vi "select elements to create channels for.vi"(8 "error in":errorcluster, 10 "allowable channels":i32[](array[numeric]), 11 "assembly definition":T1) -> (0 "error out":errorcluster, 1 "cancelled?":bool, 2 "channels to create":i32[](array[numeric]), 3 "base channame":string, 5 "create tags":bool)   [LabVIEW 2013, in "EthernetIP editor node.lvclass"]
uses:
  EthernetIP editor node.lvclass
  configuration/assembly definition.ctl
  configuration/assembly type.ctl
  <vilib>/NI/Tag Bus/tag/Data Type.ctl
  configuration/EthernetIP configuration.lvclass
  <vilib>/NI/Tag Bus/tag/tag descriptor.lvclass
panel:
  in  "Also Create Tags?":bool
  in  "cancel":bool
  in  "Base Name":string
  in  "OK":bool
  in  "Remove":bool
  in  "Add":bool
  in  "Channels to Configure":i32[](listbox)
  in  "Allowable Channels":i32[](listbox)
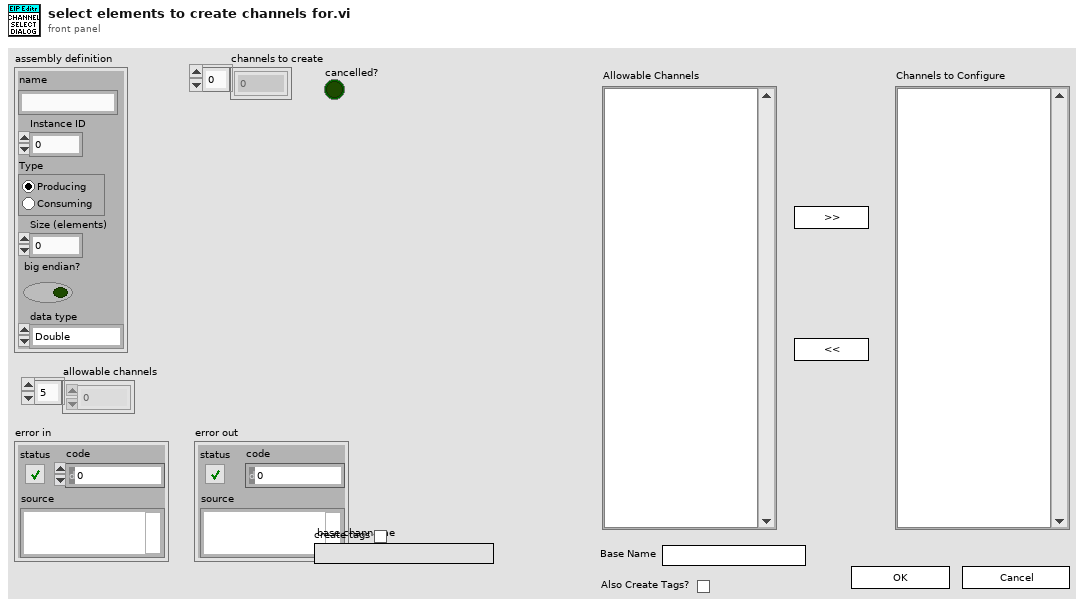
[diagram p1: front panel]
types:
  T1 = typedef "EthernetIP configuration.lvclass/assembly definition.ctl" = cluster{"name":string, "Instance ID":u32, "Type":T2, "Size (elements)":u32, "big endian?":bool, "data type":T3}
  T2 = typedef "EthernetIP configuration.lvclass/assembly type.ctl" = enum32{"Producing", "Consuming"}
  T3 = typedef "tag bus.lvlib/tag descriptor.lvclass/Data Type.ctl" = enum16{"Double", "Single", "I64", "I32", "I16", "I8", "U64", "U32", "U16", "U8", "Boolean", "String", "Array of Double", "Array of Single", "Array of I64", "Array of I32", "Array of I16", "Array of I8", "Array of U64", "Array of U32", "Array of U16", "Array of U8", "Array of Boolean", "Array of String"}
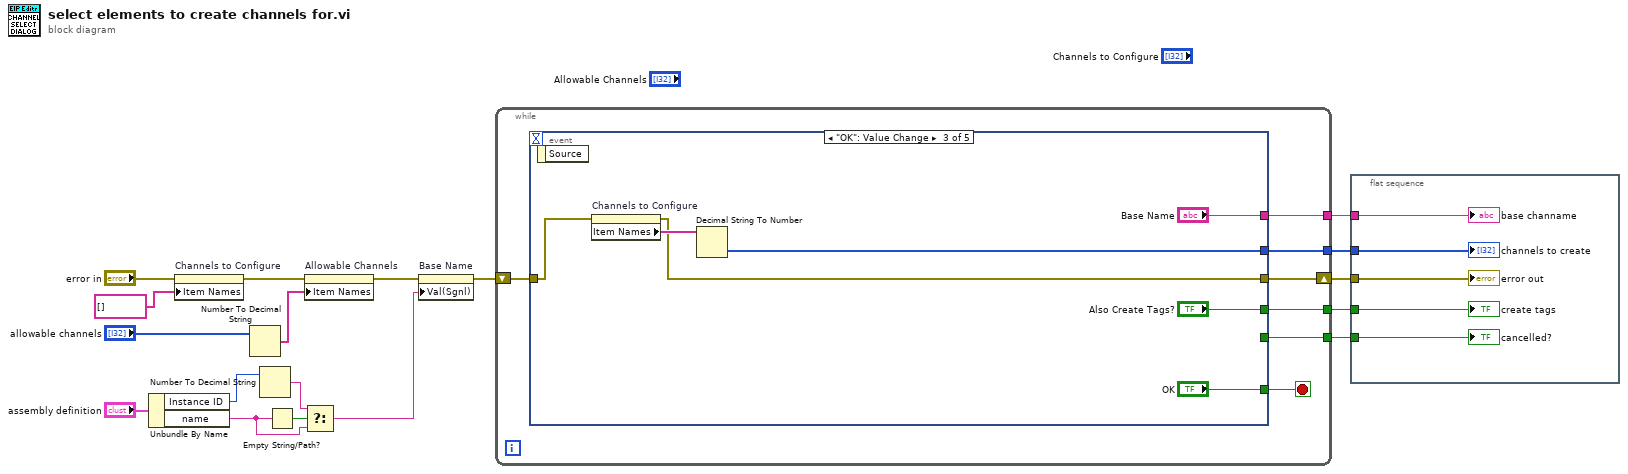
[diagram p0: block diagram]
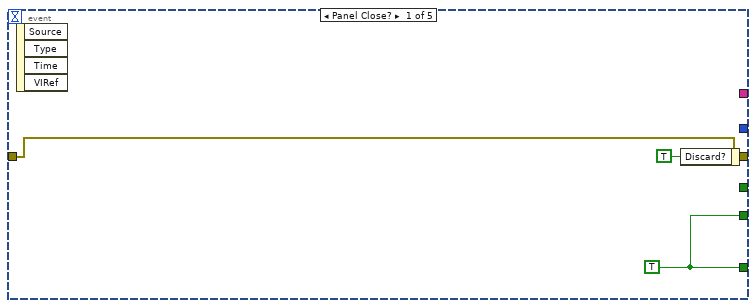
[diagram p2: hidden frame]
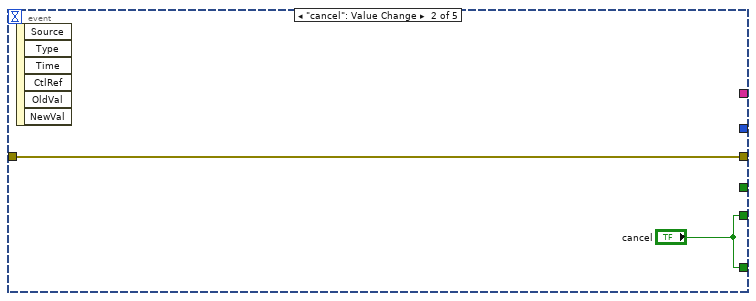
[diagram p3: hidden frame]
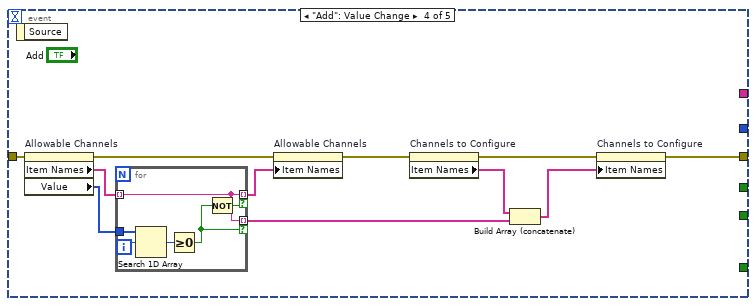
[diagram p4: hidden frame]
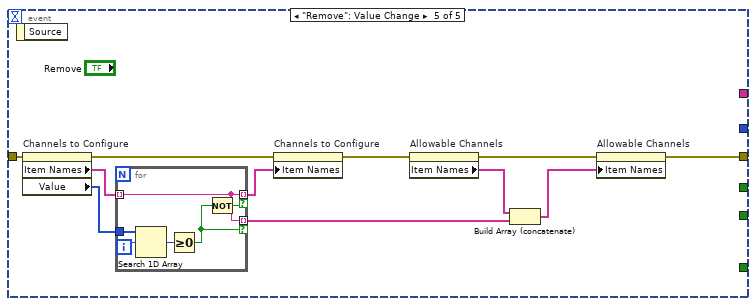
[diagram p5: hidden frame]
diagram:
  n1 = Unbundle By Name("assembly definition") -> ("Instance ID"=w8:u32, "name"=w9:string)
  n2 = property on="Channels to Configure" class="LstBox (strict)"(error in="error in", "Item Names"=string[] []) -> (error out=w4:errorcluster)  [unwired: 1 in, 1 out]
  n3 = Number To Decimal String(number="allowable channels") -> (decimal integer string=w15:string[])  [unwired: 1 in]
  n4 = Number To Decimal String(number=w8) -> (decimal integer string=w7:string)  [unwired: 1 in]
  n5 = Empty String/Path?(string/path=w9) -> (empty?=w10:bool)
  n6 = property on="Allowable Channels" class="LstBox (strict)"(error in=w4, "Item Names"=w15) -> (error out=w12:errorcluster)  [unwired: 1 in, 1 out]
  n7 = Select(t=w7, s=w10, f=w9) -> (s? t:f=w6:string)
  n8 = property on="Base Name" class="Str"(error in=w12, "Val(Sgnl)"=w6) -> (error out=w11:errorcluster)  [unwired: 1 in, 1 out]
  n9 = while {
    tunnel: [w24] -> w18
    tunnel: [w23] -> w17
    shift-right: [w21] -> w16
    shift-left: w11 -> [w22]
    tunnel: [w20] -> w5
    tunnel: [w19] -> w1
    stop <- w25 stop-if-true
    n10 = event shown="[2] \"OK\": Value Change" {
      selector: _ -> [_ _ _ _ _]
      dyn-events: _ -> [_ _ _ _ _]
      timeout: _ -> [_ _ _ _ _]
      tunnel: [w27 "cancel" "OK" _ _] -> w25
      tunnel: [w27 "cancel" _ _ _] -> w24
      tunnel: [_ _ w35 _ _] -> w23
      tunnel: w22 -> [w26 w29 w34 w48 w65]
      tunnel: [w26 w29 w33 w45 w62] -> w21
      tunnel: [_ _ "Base Name" _ _] -> w20
      tunnel: [_ _ "Also Create Tags?" _ _] -> w19
      event Panel Close? {
        w27 = TRUE
        n11 = event-data() -> ()  [unwired: 1 in, 4 out]
        n12 = event-data("Discard?"=TRUE) -> ()  [unwired: 1 in, 1 out]
      }
      event "cancel": Value Change {
        n13 = event-data() -> ()  [unwired: 1 in, 6 out]
      }
      event "OK": Value Change {
        n14 = event-data() -> ()  [unwired: 1 in, 1 out]
        n15 = property on="Channels to Configure" class="LstBox (strict)"(error in=w34) -> (error out=w33:errorcluster, "Item Names"=w36:string[])  [unwired: 1 in, 1 out]
        n16 = Decimal String To Number(string=w36) -> (number=w35:i32[])  [unwired: 2 in, 1 out]
      }
      event "Add": Value Change {
        n17 = event-data() -> ()  [unwired: 1 in, 1 out]
        n18 = property on="Allowable Channels" class="LstBox (strict)"(error in=w48) -> (error out=w47:errorcluster, "Item Names"=w43:string[], "Value"=w42:i32[])  [unwired: 1 in, 1 out]
        n19 = for {
          tunnel: w43 -> [w51] mode=indexing
          tunnel: w42 -> [w54]
          tunnel: [w51] -> w41 mode=indexing if=w50
          tunnel: [w51] -> w38 mode=indexing if=w49
          i -> [w53]
          n20 = Search 1D Array(1D array=w54, element=w53) -> (index of element=w52:i32)  [unwired: 1 in]
          n21 = Greater Or Equal To 0?(x=w52) -> (x >= 0?=w49:bool)
          n22 = Not(x=w49) -> (.not. x?=w50:bool)
        }
        n23 = property on="Allowable Channels" class="LstBox (strict)"(error in=w47, "Item Names"=w41) -> (error out=w46:errorcluster)  [unwired: 1 in, 1 out]
        n24 = property on="Channels to Configure" class="LstBox (strict)"(error in=w46) -> (error out=w44:errorcluster, "Item Names"=w40:string[])  [unwired: 1 in, 1 out]
        n25 = Build Array (concatenate)(w40, w38) -> (w39:string[])
        n26 = property on="Channels to Configure" class="LstBox (strict)"(error in=w44, "Item Names"=w39) -> (error out=w45:errorcluster)  [unwired: 1 in, 1 out]
      }
      event "Remove": Value Change {
        n27 = event-data() -> ()  [unwired: 1 in, 1 out]
        n28 = property on="Channels to Configure" class="LstBox (strict)"(error in=w65) -> (error out=w64:errorcluster, "Item Names"=w60:string[], "Value"=w59:i32[])  [unwired: 1 in, 1 out]
        n29 = for {
          tunnel: w60 -> [w68] mode=indexing
          tunnel: w59 -> [w71]
          tunnel: [w68] -> w58 mode=indexing if=w67
          tunnel: [w68] -> w55 mode=indexing if=w66
          i -> [w70]
          n30 = Search 1D Array(1D array=w71, element=w70) -> (index of element=w69:i32)  [unwired: 1 in]
          n31 = Greater Or Equal To 0?(x=w69) -> (x >= 0?=w66:bool)
          n32 = Not(x=w66) -> (.not. x?=w67:bool)
        }
        n33 = property on="Channels to Configure" class="LstBox (strict)"(error in=w64, "Item Names"=w58) -> (error out=w63:errorcluster)  [unwired: 1 in, 1 out]
        n34 = property on="Allowable Channels" class="LstBox (strict)"(error in=w63) -> (error out=w61:errorcluster, "Item Names"=w57:string[])  [unwired: 1 in, 1 out]
        n35 = Build Array (concatenate)(w57, w55) -> (w56:string[])
        n36 = property on="Allowable Channels" class="LstBox (strict)"(error in=w61, "Item Names"=w56) -> (error out=w62:errorcluster)  [unwired: 1 in, 1 out]
      }
    }
  }
  n37 = flat-sequence {
    tunnel: w18 -> [w76]
    tunnel: w17 -> [w75]
    tunnel: w16 -> [w74]
    tunnel: w5 -> [w73]
    tunnel: w1 -> [w72]
    frame #0 {
      "channels to create" <- w75
      "error out" <- w74
      "cancelled?" <- w76
      "base channame" <- w73
      "create tags" <- w72
    }
  }
